vi "Get UI VI Reference.vi"(8 "error in (no error)":errorcluster, 11 "Flex UI in":refnum<class "Flex UI.lvclass">) -> (0 "error out":errorcluster, 2 "UI VI Reference":refnum<vi>, 3 "Flex UI out":refnum<class "Flex UI.lvclass">)   [LabVIEW 2016, in "Flex UI.lvclass"]
uses:
  Flex UI.lvclass
  Flex UI.lvclass/Flex UI.ctl
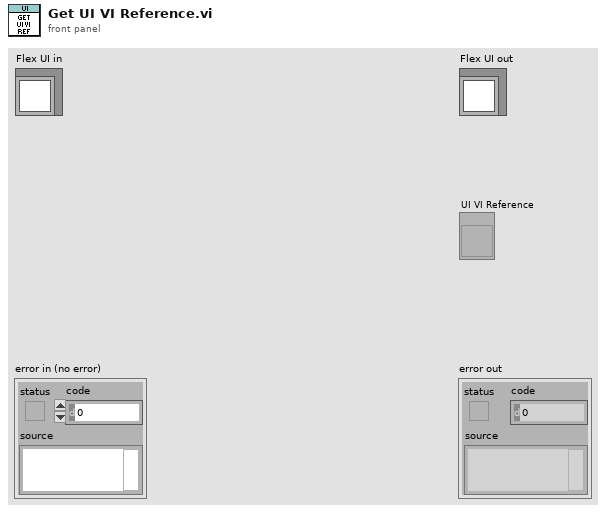
[diagram p1: front panel]
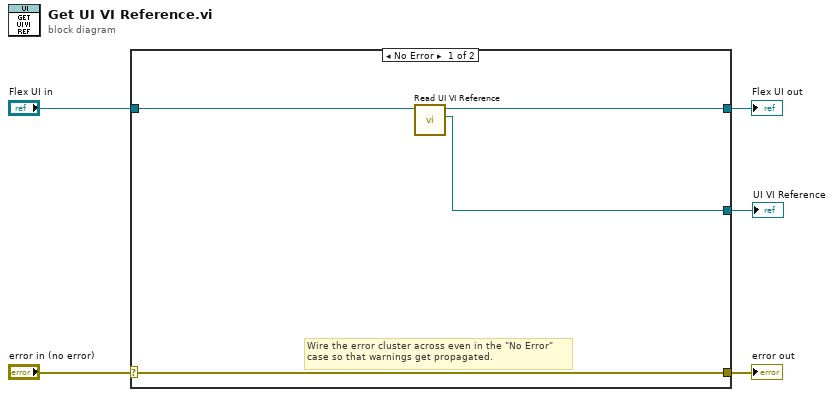
[diagram p0: block diagram]
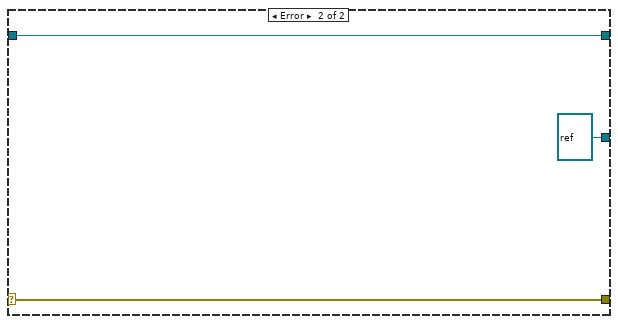
[diagram p2: hidden frame]
diagram:
  n1 = case shown="No Error" "error in (no error)" {
    selector: "error in (no error)" -> [w8 w12]
    tunnel: [w8 w12] -> w4
    tunnel: [w7 w11] -> w2
    tunnel: "Flex UI in" -> [w9 w11]
    tunnel: [w6 refnum<vi> refnum ("UI VI Reference")] -> w1
    frame No Error {
      # "Wire the error cluster across even in the \"No Error\"\ncase so that warnings get propagated."
      n2 = call "Read UI VI Reference.vi"("Flex UI in"=w9) -> ("UI VI Reference"=w6:refnum<vi>, "Flex UI out"=w7:refnum<class "Flex UI.lvclass">)  [unwired: 9 in]
    }
    frame Error {
    }
  }
  "error out" <- w4
  "Flex UI out" <- w2
  "UI VI Reference" <- w1
